vi "VG_BT3562.vi"() -> ()   [LabVIEW 2020]
panel:
  out "BT3562":string
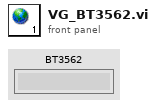
[diagram p1: front panel]
diagram:
